vi "Open TDMS.vi"(7 "Operation (0:open)":T1(ring), 8 "error in (no error)":errorcluster, 9 "File Path":path, 10 "Record Group Name":string, 11 "Sparkfun Atomic IMU in":refnum<class "Sparkfun Atomic IMU.lvclass">) -> (0 "error out":errorcluster, 3 "Sparkfun Atomic IMU out":refnum<class "Sparkfun Atomic IMU.lvclass">)   [LabVIEW 2019, in "Sparkfun Atomic IMU.lvclass"]
doc: "Opens a tdms file to record sensor data."
uses:
  Sparkfun Atomic IMU.lvclass
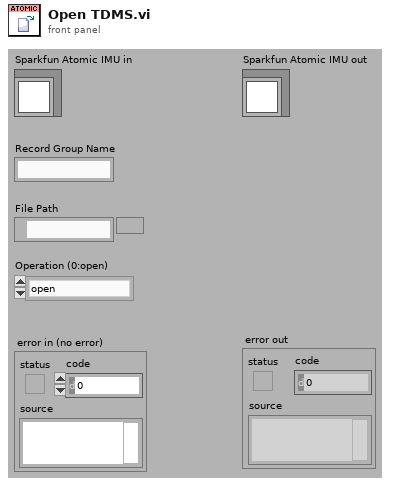
[diagram p1: front panel]
types:
  T1 = enum16{"open", "open or create", "create or replace", "create", "open (read-only)"}
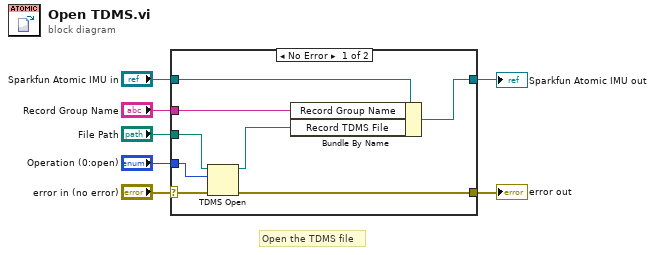
[diagram p0: block diagram]
diagram:
  # "Open the TDMS file"
  n1 = case shown="No Error" "error in (no error)" {
    selector: "error in (no error)" -> [w13 w17]
    tunnel: [w12 w17] -> w6
    tunnel: "Sparkfun Atomic IMU in" -> [w15 w16]
    tunnel: "File Path" -> [w14 _]
    tunnel: "Operation (0:open)" -> [w11 _]
    tunnel: "Record Group Name" -> [w10 _]
    tunnel: [w8 w16] -> w1
    frame No Error {
      n2 = TDMS Open(8:w13, 10:w11, 11:w14) -> (0:w12:errorcluster, 3:w9:refnum<k34>)  [unwired: 4 in]
      n3 = Bundle By Name(cluster=w15, "Record Group Name"=w10, "Record TDMS File"=w9) -> (w8:refnum<class "Sparkfun Atomic IMU.lvclass">)
    }
    frame Error {
    }
  }
  "Sparkfun Atomic IMU out" <- w1
  "error out" <- w6
